vi "Example_Set_Get Functios_StringFormat.vi"() -> ()   [LabVIEW 2020]
doc: "Demonstrates how GUI object values can be saved into configuration file or loaded from the configuration file. This feature is extremely useful to manage settings of the application. Another, and very important, feature is that adding or removing items to be saved is taking minimum time. \nThe example illustrates how to either get control/indicator value in or from string format."
uses:
  VI Server Toolkit LV2013.lvlib
  VI Server Libraries/VI Server_Set Controls.llb/Set STR Control.vi
panel:
  in  "Tab.Main":enum32{"Set/Get1", "Set/Get2"}(tab)
  in  "Menu Ring.Item Names":string[](array[string])=["Item 1", "Item 2", "Item 3"] caption="1D Array - String"
  in  "CtlValue.String":string caption="Control Value: String"
  in  "Slide.Get":bool
  in  "Slide.Set":bool
  in  "Menu Ring.Get":bool
  in  "Menu Ring.Set":bool
  in  "File Path.Get":bool
  in  "File Path.Set":bool
  in  "LED.Get":bool
  in  "LED.Set":bool
  in  "Button.Get":bool
  in  "Button.Set":bool
  in  "Knob.Get":bool
  in  "Knob.Set":bool
  in  "Numeric.Get":bool
  in  "Numeric.Set":bool
  in  "File Path.Mirror":path
  in  "Numeric.Mirror":dbl=5.0 caption="Numeric Control"
  in  "Slide.Mirror":dbl(slide)=1.9191919191919191 caption="Horizontal Fill Slide" scale=0.0..10.0
  in  "Knob.Mirror":dbl(knob) caption="Knob" scale=0.0..10.0
  in  "Button.Mirror":bool caption="Settings Button"
  in  "Menu Ring.Mirror":u16(ring) caption="Menu Ring" items=["Item 1", "Item 2", "Item 3"]
  in  "LED.Mirror":bool caption="LED"
  in  "ArrayCtlValue.String":string caption="Control Value: String"
  in  "2D Array - Boolean.Get":bool caption="2D Array - Path.Get"
  in  "2D Array - Boolean.Set":bool caption="2D Array - Path.Set"
  in  "2D Array - DBL.Get":bool
  in  "2D Array - DBL.Set":bool
  in  "1D Array - DBL.Get":bool
  in  "1D Array - DBL.Set":bool
  in  "2D Array - String.Get":bool
  in  "2D Array - String.Set":bool
  in  "1D Array - String.Mirror":string[](array[string]) caption="1D Array - String"
  in  "2D Array - String.Mirror":string[][](array[string]) caption="2D Array - String"
  in  "1D Array - DBL.Mirror":dbl[](array[numeric]) caption="1D Array - DBL"
  in  "2D Array - DBL.Mirror":dbl[][](array[numeric]) caption="2D Array - DBL"
  in  "2D Array - Path.Mirror":path[][](array[path]) caption="2D Array - String"
  in  "2D Array - Boolean.Mirror":bool[][](array[boolean]) caption="2D Array - String"
  in  "1D Array - String.Get":bool
  in  "1D Array - String.Set":bool
  in  "2D Array - Path.Get":bool
  in  "2D Array - Path.Set":bool
  in  "EXIT":bool
  in  "Error In":errorcluster
  out "error out":errorcluster
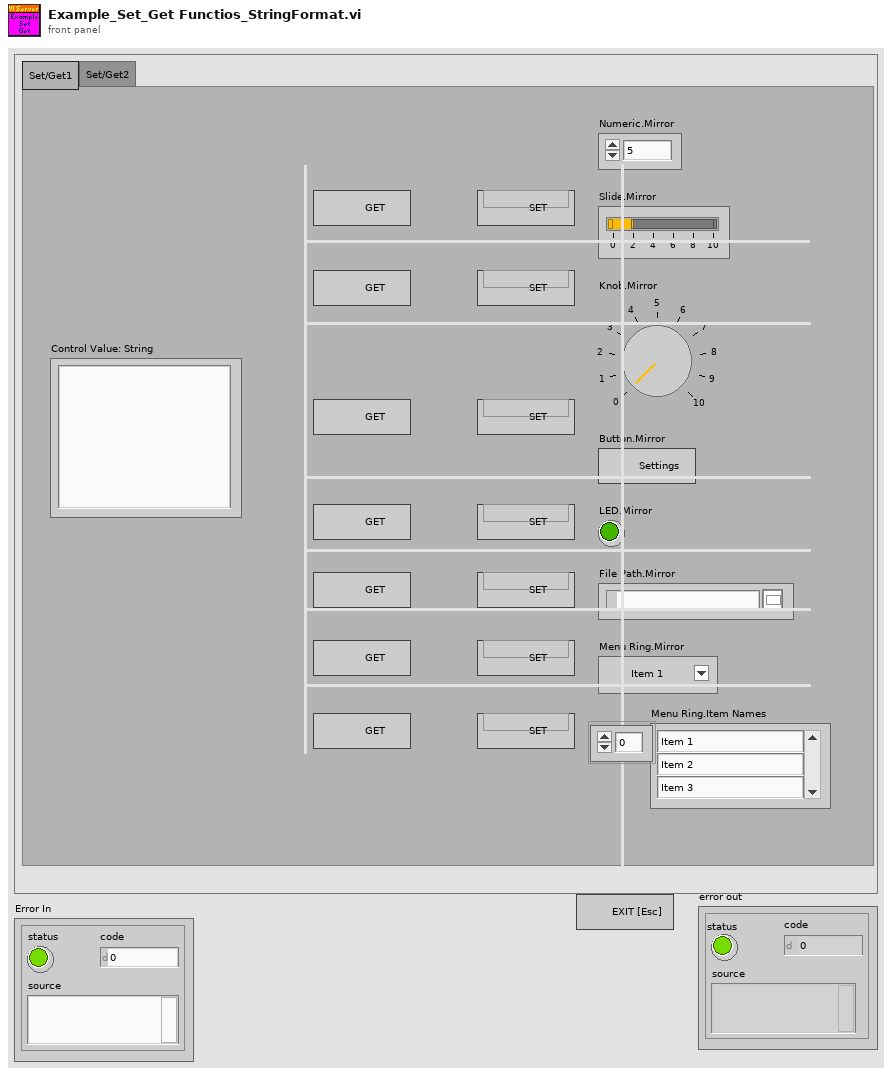
[diagram p1: front panel]
types:
  T1 = typedef "VI Server_RefsCluster.ctl" = cluster{"Labels":string[], "Refs":refnum<vi>[], "VI Ref":refnum<vi>}
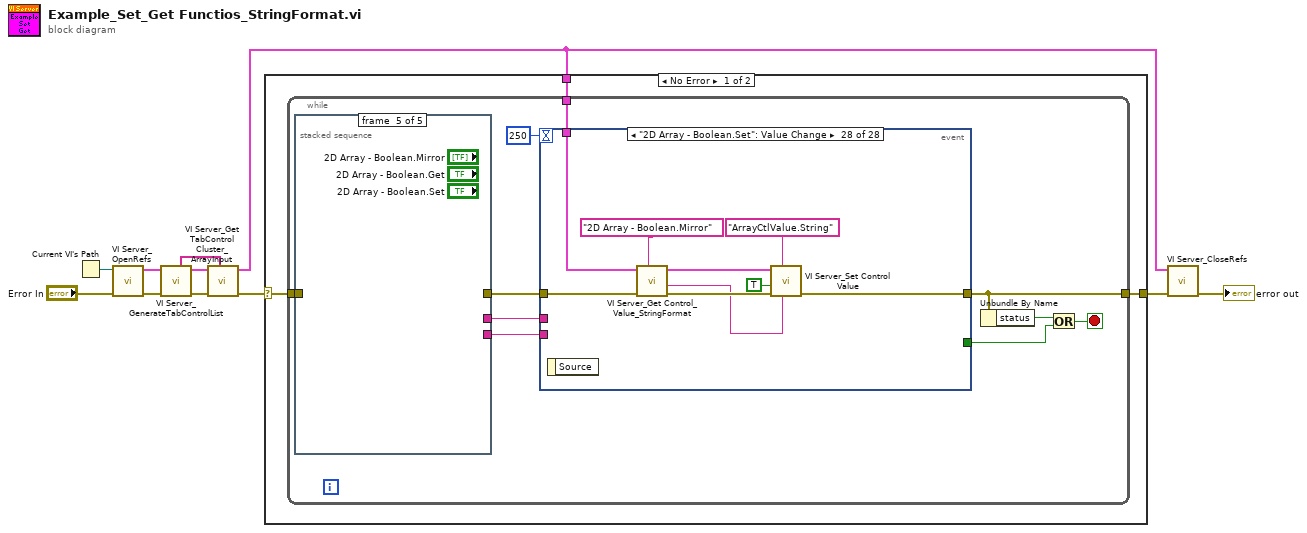
[diagram p0: block diagram]
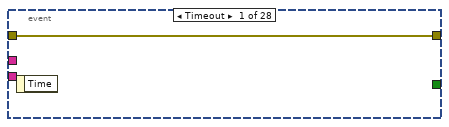
[diagram p2: hidden frame]
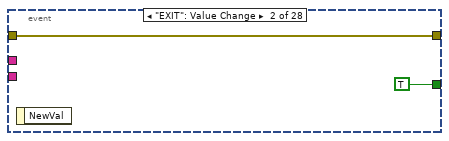
[diagram p3: hidden frame]
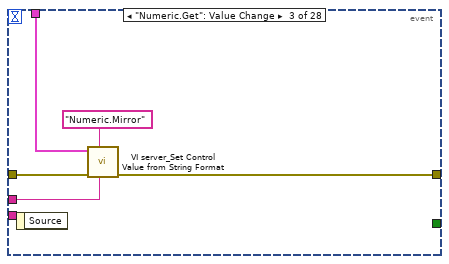
[diagram p4: hidden frame]
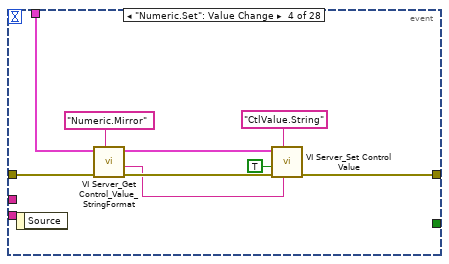
[diagram p5: hidden frame]
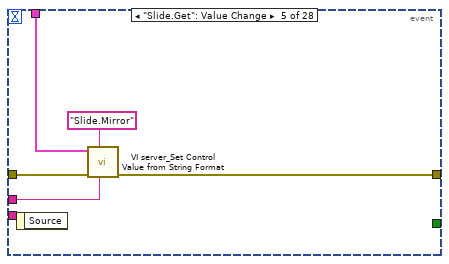
[diagram p6: hidden frame]
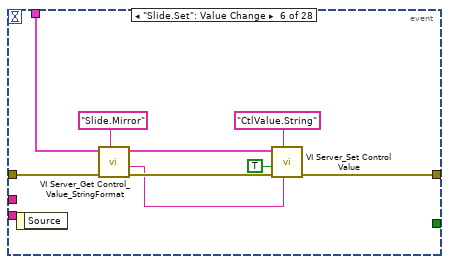
[diagram p7: hidden frame]
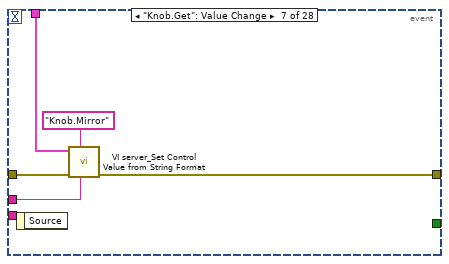
[diagram p8: hidden frame]
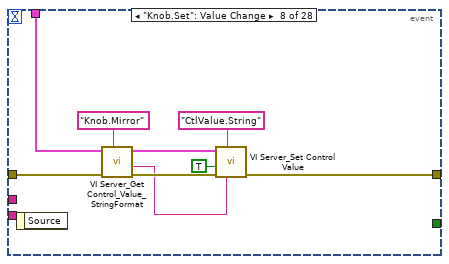
[diagram p9: hidden frame]
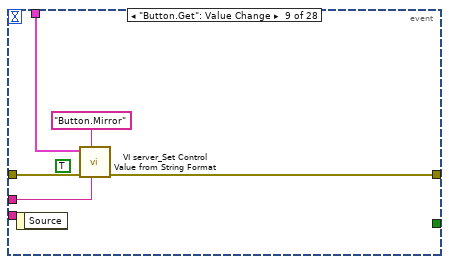
[diagram p10: hidden frame]
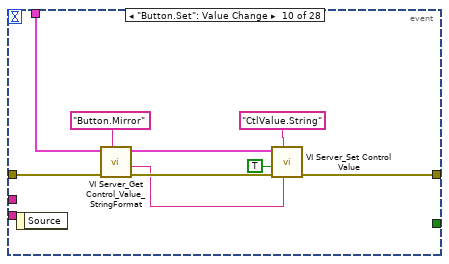
[diagram p11: hidden frame]
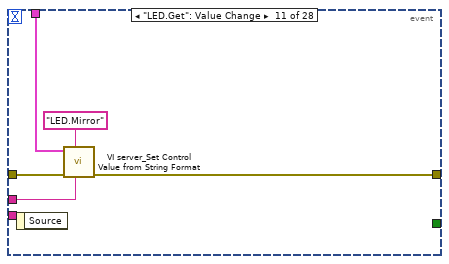
[diagram p12: hidden frame]
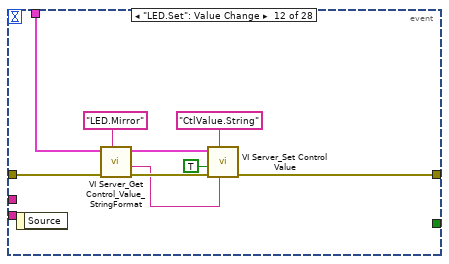
[diagram p13: hidden frame]
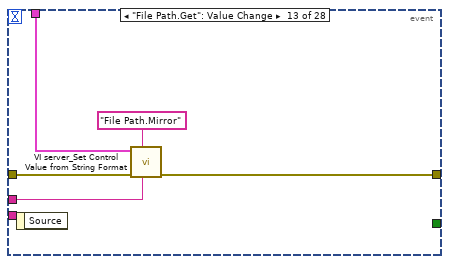
[diagram p14: hidden frame]
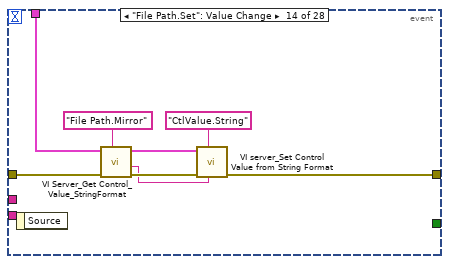
[diagram p15: hidden frame]
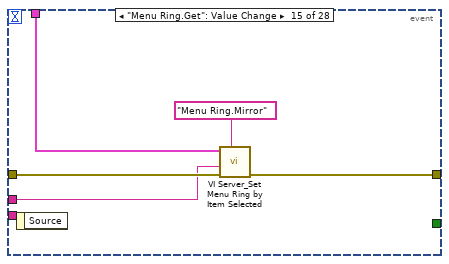
[diagram p16: hidden frame]
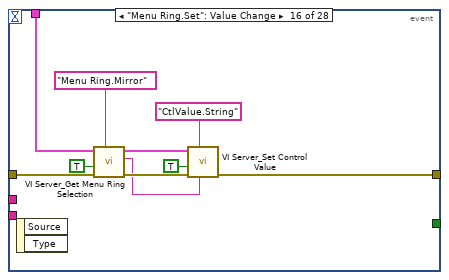
[diagram p17: hidden frame]
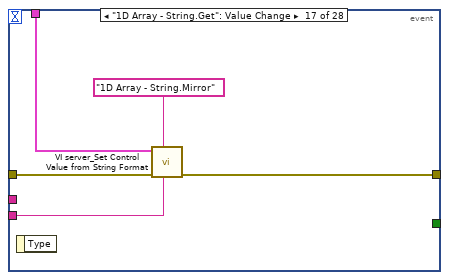
[diagram p18: hidden frame]
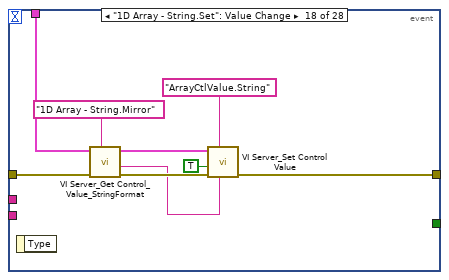
[diagram p19: hidden frame]
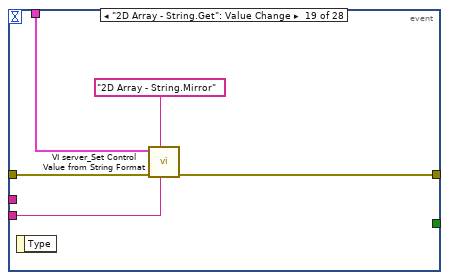
[diagram p20: hidden frame]
diagram:
  n1 = Current VI's Path() -> (path=w10:path)
  n2 = call "VI Server_OpenRefs.vi"("error in"="Error In", "VI Path"=w10) -> ("error out"=w4:errorcluster, "VI Server.RefsCluster"=w5:T1)  [unwired: 8 in]
  n3 = call "VI Server_GenerateTabControlList.vi"("error in (no error)"=w4, "VI Server Cluster"=w5) -> ("error out"=w7:errorcluster, "VI Server Cluster.DUP"=w6:T1, "TabControls"=w2:string[])  [unwired: 7 in]
  n4 = call "VI Server_Get TabControl Cluster_ArrayInput.vi"("TabControl Labels[]"=w2, "error in"=w7, "VI Server Cluster"=w6) -> ("error out"=w3:errorcluster, "VI Server Cluster.OUT"=w1:T1)  [unwired: 7 in]
  n5 = case shown="No Error" w3 {
    selector: w3 -> [w14 w213]
    tunnel: [w13 w213] -> w9
    tunnel: w1 -> [w12 _]
    frame No Error {
      n6 = while {
        tunnel: w14 -> [w23]
        tunnel: [w21] -> w13
        tunnel: w12 -> [w17]
        stop <- w18 stop-if-true
        n7 = stacked-sequence {
          tunnel: [w212 _ _ _ _] -> w22
          tunnel: w23 -> [w212 _ _ _ _]
          tunnel: ["CtlValue.String" _ _ _ _] -> w16
          tunnel: ["ArrayCtlValue.String" _ _ _ _] -> w15
          frame #0 {
          }
          frame #1 {
          }
          frame #2 {
          }
          frame #3 {
          }
          frame #4 {
          }
        }
        n8 = event shown="[27] \"2D Array - Boolean.Set\": Value Change" {
          selector: _ -> [_ _ _ _ _ _ _ _ _ _ _ _ _ _ _ _ _ _ _ _ _ _ _ _ _ _ _ _]
          dyn-events: _ -> [_ _ _ _ _ _ _ _ _ _ _ _ _ _ _ _ _ _ _ _ _ _ _ _ _ _ _ _]
          timeout: 250 -> [_ _ _ _ _ _ _ _ _ _ _ _ _ _ _ _ _ _ _ _ _ _ _ _ _ _ _ _]
          tunnel: w22 -> [w25 w27 w30 w38 w44 w50 w60 w66 w72 w83 w84 w97 w100 w110 w114 w122 w128 w139 w142 w153 w156 w167 w172 w181 w184 w195 w199 w203]
          tunnel: [w25 w27 w32 w41 w46 w55 w58 w69 w74 w79 w88 w93 w102 w106 w113 w120 w130 w133 w144 w147 w158 w161 w171 w175 w186 w189 w198 w201] -> w21
          tunnel: [_ TRUE _ _ _ _ _ _ _ _ _ _ _ _ _ _ _ _ _ _ _ _ _ _ _ _ _ _] -> w19
          tunnel: w17 -> [_ _ w29 w35 w43 w52 w59 w64 w71 w82 w85 w96 w98 w109 w112 w123 w127 w138 w141 w152 w155 w166 w169 w180 w183 w194 w197 w202]
          tunnel: w16 -> [_ _ w28 _ w42 _ w56 _ w70 _ w86 _ w99 _ w111 _ _ _ _ _ _ _ _ _ _ _ _ _]
          tunnel: w15 -> [_ _ _ _ _ _ _ _ _ _ _ _ _ _ _ _ w126 _ w140 _ w154 _ w168 _ w182 _ w196 _]
          event Timeout {
            n9 = event-data() -> ()  [unwired: 1 in, 1 out]
          }
          event "EXIT": Value Change {
            n10 = event-data() -> ()  [unwired: 1 in, 1 out]
          }
          event "Numeric.Get": Value Change {
            n11 = event-data() -> ()  [unwired: 1 in, 1 out]
            n12 = call "VI server_Set Control Value from String Format.vi"("Value.STR"=w28, "Label"="Numeric.Mirror", "error in (no error)"=w30, "VI Server Cluster"=w29) -> ("error out"=w32:errorcluster)  [unwired: 5 in, 2 out]
          }
          event "Numeric.Set": Value Change {
            n13 = event-data() -> ()  [unwired: 1 in, 1 out]
            n14 = call "VI Server_Get Control_Value_StringFormat.vi"("Label"="Numeric.Mirror", "error in (no error)"=w38, "VI Server Cluster"=w35) -> ("error out"=w37:errorcluster, "ControlValue(StringFormat)"=w34:string, "VI Server Cluster.DUP"=w33:T1)  [unwired: 5 in, 1 out]
            n15 = call-poly "VI Server_Set Control Value.vi"("New Value"=w34, "Label"="CtlValue.String", "error in"=w37, "Single Instance (T)"=TRUE, "VI Server Cluster"=w33) -> ("error out"=w41:errorcluster)  [unwired: 4 in, 2 out]
          }
          event "Slide.Get": Value Change {
            n16 = event-data() -> ()  [unwired: 1 in, 1 out]
            n17 = call "VI server_Set Control Value from String Format.vi"("Value.STR"=w42, "Label"="Slide.Mirror", "error in (no error)"=w44, "VI Server Cluster"=w43) -> ("error out"=w46:errorcluster)  [unwired: 5 in, 2 out]
          }
          event "Slide.Set": Value Change {
            n18 = event-data() -> ()  [unwired: 1 in, 1 out]
            n19 = call "VI Server_Get Control_Value_StringFormat.vi"("Label"="Slide.Mirror", "error in (no error)"=w50, "VI Server Cluster"=w52) -> ("error out"=w49:errorcluster, "ControlValue(StringFormat)"=w47:string, "VI Server Cluster.DUP"=w51:T1)  [unwired: 5 in, 1 out]
            n20 = call-poly "VI Server_Set Control Value.vi"("New Value"=w47, "Label"="CtlValue.String", "error in"=w49, "Single Instance (T)"=TRUE, "VI Server Cluster"=w51) -> ("error out"=w55:errorcluster)  [unwired: 4 in, 2 out]
          }
          event "Knob.Get": Value Change {
            n21 = event-data() -> ()  [unwired: 1 in, 1 out]
            n22 = call "VI server_Set Control Value from String Format.vi"("Value.STR"=w56, "Label"="Knob.Mirror", "error in (no error)"=w60, "VI Server Cluster"=w59) -> ("error out"=w58:errorcluster)  [unwired: 5 in, 2 out]
          }
          event "Knob.Set": Value Change {
            n23 = event-data() -> ()  [unwired: 1 in, 1 out]
            n24 = call "VI Server_Get Control_Value_StringFormat.vi"("Label"="Knob.Mirror", "error in (no error)"=w66, "VI Server Cluster"=w64) -> ("error out"=w65:errorcluster, "ControlValue(StringFormat)"=w61:string, "VI Server Cluster.DUP"=w63:T1)  [unwired: 5 in, 1 out]
            n25 = call-poly "VI Server_Set Control Value.vi"("New Value"=w61, "Label"="CtlValue.String", "error in"=w65, "Single Instance (T)"=TRUE, "VI Server Cluster"=w63) -> ("error out"=w69:errorcluster)  [unwired: 4 in, 2 out]
          }
          event "Button.Get": Value Change {
            (unwired) TRUE ("Single Instance (T)")
            n26 = event-data() -> ()  [unwired: 1 in, 1 out]
            n27 = call "VI server_Set Control Value from String Format.vi"("Value.STR"=w70, "Label"="Button.Mirror", "error in (no error)"=w72, "VI Server Cluster"=w71) -> ("error out"=w74:errorcluster)  [unwired: 5 in, 2 out]
          }
          event "Button.Set": Value Change {
            n28 = event-data() -> ()  [unwired: 1 in, 1 out]
            n29 = call "VI Server_Get Control_Value_StringFormat.vi"("Label"="Button.Mirror", "error in (no error)"=w83, "VI Server Cluster"=w82) -> ("error out"=w80:errorcluster, "ControlValue(StringFormat)"=w76:string, "VI Server Cluster.DUP"=w77:T1)  [unwired: 5 in, 1 out]
            n30 = call-poly "VI Server_Set Control Value.vi"("New Value"=w76, "Label"="CtlValue.String", "error in"=w80, "Single Instance (T)"=TRUE, "VI Server Cluster"=w77) -> ("error out"=w79:errorcluster)  [unwired: 4 in, 2 out]
          }
          event "LED.Get": Value Change {
            n31 = event-data() -> ()  [unwired: 1 in, 1 out]
            n32 = call "VI server_Set Control Value from String Format.vi"("Value.STR"=w86, "Label"="LED.Mirror", "error in (no error)"=w84, "VI Server Cluster"=w85) -> ("error out"=w88:errorcluster)  [unwired: 5 in, 2 out]
          }
          event "LED.Set": Value Change {
            n33 = event-data() -> ()  [unwired: 1 in, 1 out]
            n34 = call "VI Server_Get Control_Value_StringFormat.vi"("Label"="LED.Mirror", "error in (no error)"=w97, "VI Server Cluster"=w96) -> ("error out"=w94:errorcluster, "ControlValue(StringFormat)"=w90:string, "VI Server Cluster.DUP"=w91:T1)  [unwired: 5 in, 1 out]
            n35 = call-poly "VI Server_Set Control Value.vi"("New Value"=w90, "Label"="CtlValue.String", "error in"=w94, "Single Instance (T)"=TRUE, "VI Server Cluster"=w91) -> ("error out"=w93:errorcluster)  [unwired: 4 in, 2 out]
          }
          event "File Path.Get": Value Change {
            n36 = event-data() -> ()  [unwired: 1 in, 1 out]
            n37 = call "VI server_Set Control Value from String Format.vi"("Value.STR"=w99, "Label"="File Path.Mirror", "error in (no error)"=w100, "VI Server Cluster"=w98) -> ("error out"=w102:errorcluster)  [unwired: 5 in, 2 out]
          }
          event "File Path.Set": Value Change {
            n38 = event-data() -> ()  [unwired: 1 in, 1 out]
            n39 = call "VI Server_Get Control_Value_StringFormat.vi"("Label"="File Path.Mirror", "error in (no error)"=w110, "VI Server Cluster"=w109) -> ("error out"=w107:errorcluster, "ControlValue(StringFormat)"=w103:string, "VI Server Cluster.DUP"=w104:T1)  [unwired: 5 in, 1 out]
            n40 = call "VI server_Set Control Value from String Format.vi"("Value.STR"=w103, "Label"="CtlValue.String", "error in (no error)"=w107, "VI Server Cluster"=w104) -> ("error out"=w106:errorcluster)  [unwired: 5 in, 2 out]
          }
          event "Menu Ring.Get": Value Change {
            n41 = event-data() -> ()  [unwired: 1 in, 1 out]
            n42 = call "VI Server_Set Menu Ring by Item Selected.vi"("Label"="Menu Ring.Mirror", "error in"=w114, "Item"=w111, "VI Server Cluster"=w112) -> ("error out"=w113:errorcluster)  [unwired: 5 in, 2 out]
          }
          event "Menu Ring.Set": Value Change {
            n43 = event-data() -> ()  [unwired: 1 in, 2 out]
            n44 = call "VI Server_Get Menu Ring Selection.vi"("Label"="Menu Ring.Mirror", "error in"=w122, "Single Instance (T)"=TRUE, "VI Server Cluster"=w123) -> ("error out"=w121:errorcluster, "Selection"=w117:string, "VI Server Cluster.DUP"=w119:T1)  [unwired: 2 in, 3 out]
            n45 = call-poly "VI Server_Set Control Value.vi"("New Value"=w117, "Label"="CtlValue.String", "error in"=w121, "Single Instance (T)"=TRUE, "VI Server Cluster"=w119) -> ("error out"=w120:errorcluster)  [unwired: 4 in, 2 out]
          }
          event "1D Array - String.Get": Value Change {
            n46 = event-data() -> ()  [unwired: 1 in, 1 out]
            n47 = call "VI server_Set Control Value from String Format.vi"("Value.STR"=w126, "Label"="1D Array - String.Mirror", "error in (no error)"=w128, "VI Server Cluster"=w127) -> ("error out"=w130:errorcluster)  [unwired: 5 in, 2 out]
          }
          event "1D Array - String.Set": Value Change {
            n48 = event-data() -> ()  [unwired: 1 in, 1 out]
            n49 = call "VI Server_Get Control_Value_StringFormat.vi"("Label"="1D Array - String.Mirror", "error in (no error)"=w139, "VI Server Cluster"=w138) -> ("error out"=w136:errorcluster, "ControlValue(StringFormat)"=w131:string, "VI Server Cluster.DUP"=w135:T1)  [unwired: 5 in, 1 out]
            n50 = call-poly "VI Server_Set Control Value.vi"("New Value"=w131, "Label"="ArrayCtlValue.String", "error in"=w136, "Single Instance (T)"=TRUE, "VI Server Cluster"=w135) -> ("error out"=w133:errorcluster)  [unwired: 4 in, 2 out]
          }
          event "2D Array - String.Get": Value Change {
            n51 = event-data() -> ()  [unwired: 1 in, 1 out]
            n52 = call "VI server_Set Control Value from String Format.vi"("Value.STR"=w140, "Label"="2D Array - String.Mirror", "error in (no error)"=w142, "VI Server Cluster"=w141) -> ("error out"=w144:errorcluster)  [unwired: 5 in, 2 out]
          }
          event "2D Array - String.Set": Value Change {
            n53 = event-data() -> ()  [unwired: 1 in, 1 out]
            n54 = call "VI Server_Get Control_Value_StringFormat.vi"("Label"="2D Array - String.Mirror", "error in (no error)"=w153, "VI Server Cluster"=w152) -> ("error out"=w150:errorcluster, "ControlValue(StringFormat)"=w146:string, "VI Server Cluster.DUP"=w149:T1)  [unwired: 5 in, 1 out]
            n55 = call-poly "VI Server_Set Control Value.vi"("New Value"=w146, "Label"="ArrayCtlValue.String", "error in"=w150, "Single Instance (T)"=TRUE, "VI Server Cluster"=w149) -> ("error out"=w147:errorcluster)  [unwired: 4 in, 2 out]
          }
          event "1D Array - DBL.Get": Value Change {
            n56 = event-data() -> ()  [unwired: 1 in, 1 out]
            n57 = call "VI server_Set Control Value from String Format.vi"("Value.STR"=w154, "Label"="1D Array - DBL.Mirror", "error in (no error)"=w156, "VI Server Cluster"=w155) -> ("error out"=w158:errorcluster)  [unwired: 5 in, 2 out]
          }
          event "1D Array - DBL.Set": Value Change {
            n58 = event-data() -> ()  [unwired: 1 in, 1 out]
            n59 = call "VI Server_Get Control_Value_StringFormat.vi"("Label"="1D Array - DBL.Mirror", "error in (no error)"=w167, "VI Server Cluster"=w166) -> ("error out"=w164:errorcluster, "ControlValue(StringFormat)"=w160:string, "VI Server Cluster.DUP"=w163:T1)  [unwired: 5 in, 1 out]
            n60 = call-poly "VI Server_Set Control Value.vi"("New Value"=w160, "Label"="ArrayCtlValue.String", "error in"=w164, "Single Instance (T)"=TRUE, "VI Server Cluster"=w163) -> ("error out"=w161:errorcluster)  [unwired: 4 in, 2 out]
          }
          event "2D Array - DBL.Get": Value Change {
            n61 = event-data() -> ()  [unwired: 1 in, 1 out]
            n62 = call "VI server_Set Control Value from String Format.vi"("Value.STR"=w168, "Label"="2D Array - DBL.Mirror", "error in (no error)"=w172, "VI Server Cluster"=w169) -> ("error out"=w171:errorcluster)  [unwired: 5 in, 2 out]
          }
          event "2D Array - DBL.Set": Value Change {
            n63 = event-data() -> ()  [unwired: 1 in, 1 out]
            n64 = call "VI Server_Get Control_Value_StringFormat.vi"("Label"="2D Array - DBL.Mirror", "error in (no error)"=w181, "VI Server Cluster"=w180) -> ("error out"=w178:errorcluster, "ControlValue(StringFormat)"=w174:string, "VI Server Cluster.DUP"=w177:T1)  [unwired: 5 in, 1 out]
            n65 = call-poly "VI Server_Set Control Value.vi"("New Value"=w174, "Label"="ArrayCtlValue.String", "error in"=w178, "Single Instance (T)"=TRUE, "VI Server Cluster"=w177) -> ("error out"=w175:errorcluster)  [unwired: 4 in, 2 out]
          }
          event "2D Array - Path.Get": Value Change {
            n66 = event-data() -> ()  [unwired: 1 in, 1 out]
            n67 = call "VI server_Set Control Value from String Format.vi"("Value.STR"=w182, "Label"="2D Array - Path.Mirror", "error in (no error)"=w184, "VI Server Cluster"=w183) -> ("error out"=w186:errorcluster)  [unwired: 5 in, 2 out]
          }
          event "2D Array - Path.Set": Value Change {
            n68 = event-data() -> ()  [unwired: 1 in, 1 out]
            n69 = call "VI Server_Get Control_Value_StringFormat.vi"("Label"="2D Array - Path.Mirror", "error in (no error)"=w195, "VI Server Cluster"=w194) -> ("error out"=w192:errorcluster, "ControlValue(StringFormat)"=w188:string, "VI Server Cluster.DUP"=w191:T1)  [unwired: 5 in, 1 out]
            n70 = call-poly "VI Server_Set Control Value.vi"("New Value"=w188, "Label"="ArrayCtlValue.String", "error in"=w192, "Single Instance (T)"=TRUE, "VI Server Cluster"=w191) -> ("error out"=w189:errorcluster)  [unwired: 4 in, 2 out]
          }
          event "2D Array - Boolean.Get": Value Change {
            n71 = event-data() -> ()  [unwired: 1 in, 1 out]
            n72 = call "VI server_Set Control Value from String Format.vi"("Value.STR"=w196, "Label"="2D Array - Boolean.Mirror", "error in (no error)"=w199, "VI Server Cluster"=w197) -> ("error out"=w198:errorcluster)  [unwired: 5 in, 2 out]
          }
          event "2D Array - Boolean.Set": Value Change {
            n73 = event-data() -> ()  [unwired: 1 in, 1 out]
            n74 = call "VI Server_Get Control_Value_StringFormat.vi"("Label"="2D Array - Boolean.Mirror", "error in (no error)"=w203, "VI Server Cluster"=w202) -> ("error out"=w208:errorcluster, "ControlValue(StringFormat)"=w205:string, "VI Server Cluster.DUP"=w207:T1)  [unwired: 5 in, 1 out]
            n75 = call-poly "VI Server_Set Control Value.vi"("New Value"=w205, "Label"="ArrayCtlValue.String", "error in"=w208, "Single Instance (T)"=TRUE, "VI Server Cluster"=w207) -> ("error out"=w201:errorcluster)  [unwired: 4 in, 2 out]
          }
        }
        n76 = Unbundle By Name(w21) -> ("status"=w20:bool)
        n77 = Or(x=w20, y=w19) -> (x .or. y?=w18:bool)
      }
    }
    frame Error {
    }
  }
  n78 = call "VI Server_CloseRefs.vi"("error in"=w9, "VI Server.RefsCluster"=w1) -> ("error out"=→"error out":errorcluster)  [unwired: 9 in]
